vi "Read-Write-Settings.vi"(6 "appended array 4":refnum<vi>[][](array[refnum]), 7 "Write":bool) -> ()   [LabVIEW 2015]
uses:
  <vilib>/Rock Robotics/Network Tables/NT Write Numeric Array.vi
  <vilib>/Rock Robotics/Network Tables/NT Write Boolean.vi
panel:
  in  "Numeric":dbl
  out "millisecond timer value":u32
  in  "error in":errorcluster
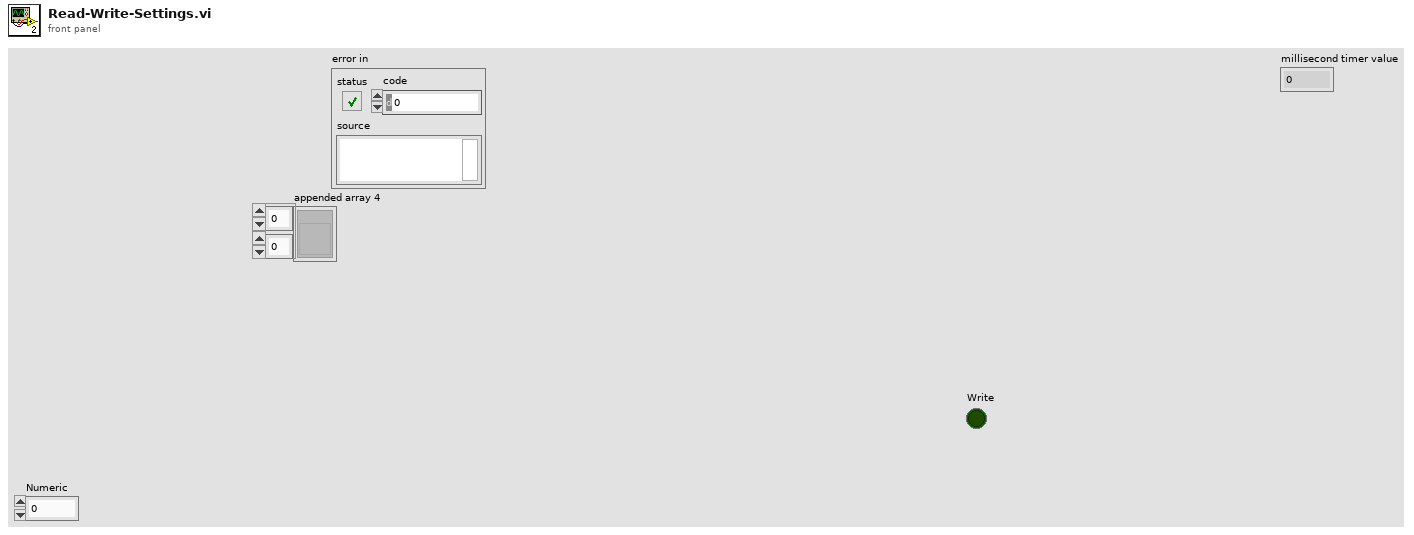
[diagram p1: front panel]
types:
  T1 = enum16{"open", "replace", "create", "open or create", "replace or create", "replace or create with confirmation"}
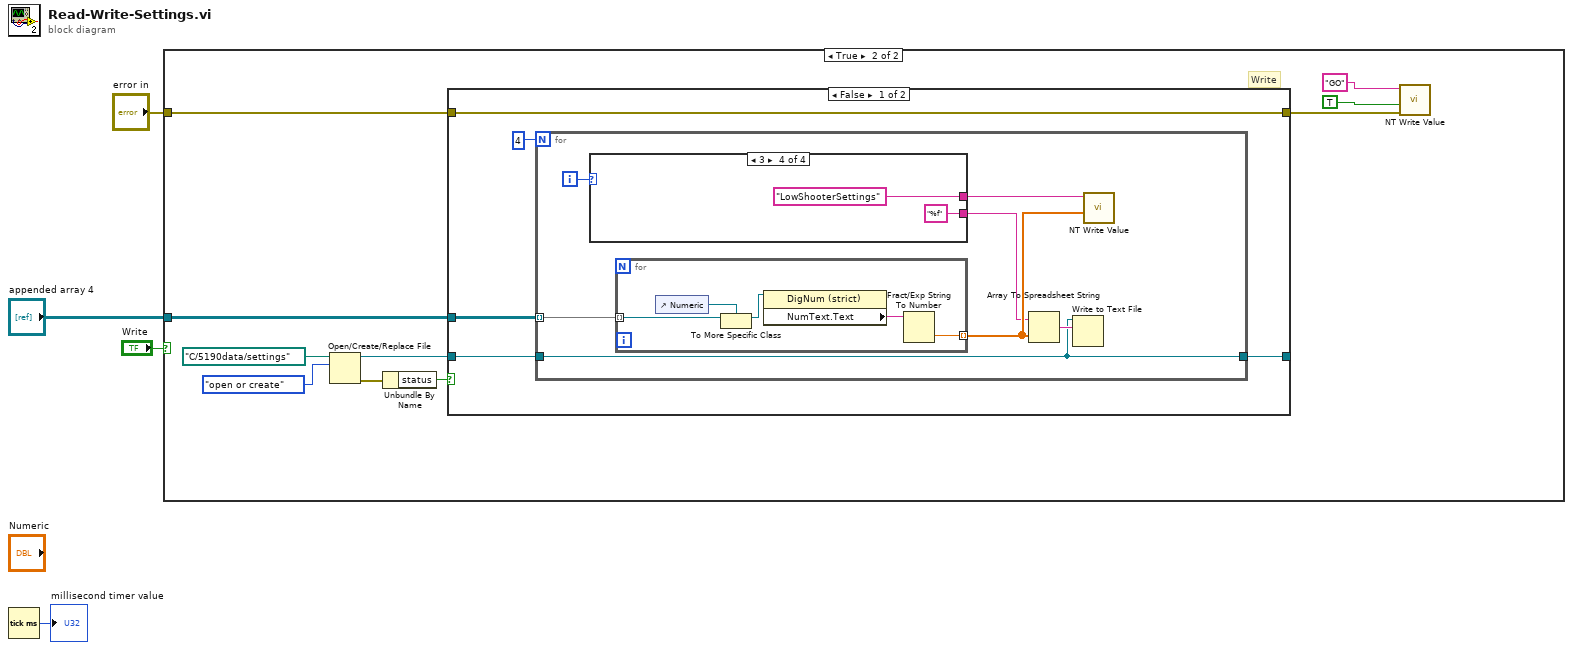
[diagram p0: block diagram]
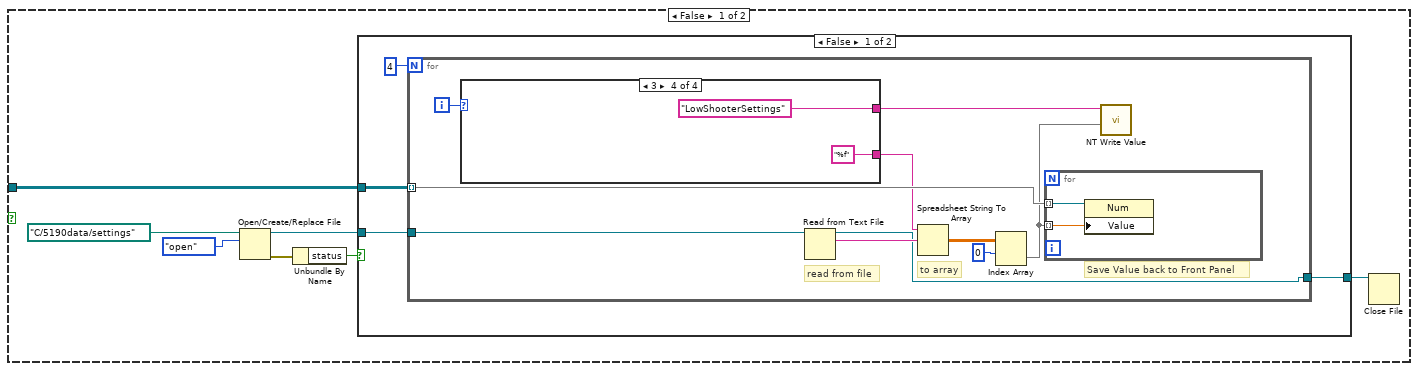
[diagram p2: hidden frame]
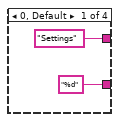
[diagram p3: hidden frame]
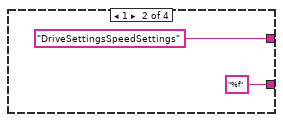
[diagram p4: hidden frame]
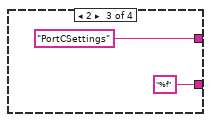
[diagram p5: hidden frame]
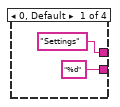
[diagram p7: hidden frame]
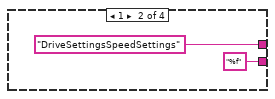
[diagram p8: hidden frame]
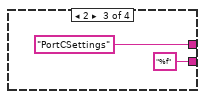
[diagram p9: hidden frame]
diagram:
  n1 = Tick Count (ms)() -> (millisecond timer value=→"millisecond timer value":u32)
  n2 = case shown="True" "Write" {
    tunnel: "error in" -> [_ w39]
    tunnel: "appended array 4" -> [w5 w37]
    frame False {
      n3 = Open/Create/Replace File(file path (use dialog)=path "C:/5190data/settings", operation (0:open)=T1."open") -> (refnum out=w7:refnum<file>, error out=w9:errorcluster)  [unwired: 4 in, 1 out]
      n4 = Unbundle By Name(w9) -> ("status"=w8:bool)
      n5 = case shown="False" w8 {
        tunnel: w7 -> [w15 w36]
        tunnel: [w13 w36] -> w6
        tunnel: w5 -> [w12 _]
        frame False {
          n6 = for {
            N: 4 -> [_]
            tunnel: w15 -> [w20]
            tunnel: [w22] -> w13
            tunnel: w12 -> [w18] mode=indexing
            i -> [w19]
            # "Save Value back to Front Panel"
            # "to array"
            # "read from file"
            n7 = case shown="3" w19 {
              tunnel: ["Settings" ("Name") "DriveSettingsSpeedSettings" ("Name") "PortCSettings" ("Name") "LowShooterSettings" ("Name")] -> w21
              tunnel: ["%d" ("format string") "%f" ("format string") "%f" ("format string") "%f" ("format string")] -> w16
              frame 0, Default {
              }
              frame 1 {
              }
              frame 2 {
              }
              frame 3 {
              }
            }
            n8 = Read from Text File(file (use dialog)=w20) -> (refnum out=w22:refnum<file>, text=w25:string)  [unwired: 3 in, 2 out]
            n9 = Spreadsheet String To Array(format string=w16, spreadsheet string=w25) -> (array=w23:dbl[][])  [unwired: 2 in]
            n10 = Index Array(array=w23, index (row)=0) -> (element=w17:dbl[])  [unwired: 1 in]
            n11 = for {
              tunnel: w18 -> [w27] mode=indexing
              tunnel: w17 -> [w26] mode=indexing
              n12 = property class="Num"(reference=w27, "Value"=w26) -> ()  [unwired: 1 in, 2 out]
            }
            n13 = call-poly <vilib>:"NT Write Value.vi"("Numeric Array"=w17, "Name"=w21) -> ()  [unwired: 9 in, 1 out]
          }
        }
        frame True {
          # "Error"
        }
      }
      n14 = Close File(refnum=w6) -> ()  [unwired: 1 in, 2 out]
    }
    frame True {
      # "Write"
      n15 = Open/Create/Replace File(file path (use dialog)=path "C:/5190data/settings", operation (0:open)=T1."open or create") -> (refnum out=w42:refnum<file>, error out=w44:errorcluster)  [unwired: 4 in, 1 out]
      n16 = Unbundle By Name(w44) -> ("status"=w43:bool)
      n17 = case shown="False" w43 {
        tunnel: w42 -> [w50 w73]
        tunnel: [w49 w73] -> _
        tunnel: [w48 w72] -> w38
        tunnel: w39 -> [w48 w72]
        tunnel: w37 -> [w47 _]
        frame False {
          n18 = for {
            N: 4 -> [_]
            tunnel: w50 -> [w56]
            tunnel: [w56] -> w49
            tunnel: w47 -> [w53] mode=indexing
            i -> [w55]
            n19 = case shown="3" w55 {
              tunnel: ["Settings" ("Name") "DriveSettingsSpeedSettings" ("Name") "PortCSettings" ("Name") "LowShooterSettings" ("Name")] -> w57
              tunnel: ["%d" ("format string") "%f" ("format string") "%f" ("format string") "%f" ("format string")] -> w52
              frame 0, Default {
              }
              frame 1 {
              }
              frame 2 {
              }
              frame 3 {
              }
            }
            n20 = for {
              tunnel: w53 -> [w62] mode=indexing
              tunnel: [w63] -> w54 mode=indexing
              n21 = control-ref of="Numeric"() -> (w61:refnum<vi>)
              n22 = To More Specific Class(target class=w61, reference=w62) -> (specific class reference=w60:refnum<vi>)  [unwired: 1 in, 1 out]
              n23 = property class="DigNum (strict)"(reference=w60) -> ("NumText.Text"=w59:string)  [unwired: 1 in, 2 out]
              n24 = Fract/Exp String To Number(string=w59) -> (number=w63:dbl)  [unwired: 3 in, 1 out]
            }
            n25 = Array To Spreadsheet String(array=w54, 3:w52) -> (spreadsheet string=w58:string)  [unwired: 1 in]
            n26 = Write to Text File(file (use dialog)=w56, text=w58) -> ()  [unwired: 1 in, 4 out]
            n27 = call-poly <vilib>:"NT Write Value.vi"("Numeric Array"=w54, "Name"=w57) -> ()  [unwired: 9 in, 1 out]
          }
        }
        frame True {
        }
      }
      n28 = call-poly <vilib>:"NT Write Value.vi"("error in"=w38, "Boolean"=TRUE, "Name"="GO") -> ()  [unwired: 8 in, 1 out]
    }
  }
